vi "File or directory exists.vi"(8 "error in (no error)":errorcluster, 10 "Path":string, 11 "FTP in":refnum<class "FTP.lvclass">) -> (0 "error out":errorcluster, 1 "Exists?":bool, 2 "Path out (dup)":string, 3 "FTP out":refnum<class "FTP.lvclass">, 4 "Type":T1)   [LabVIEW 2015, in "RT Management.lvlib" / "FTP.lvclass"]
uses:
  FTP.lvclass
  File Transfer Behavior/Type.ctl
  FTP.lvclass/FTP.ctl
  Get Session.vi
  <vilib>/Utility/error.llb/Trim Whitespace.vi
  File Transfer Behavior/File Transfer Behavior.lvclass
  <vilib>/FTP/NI_FTP.lvlib
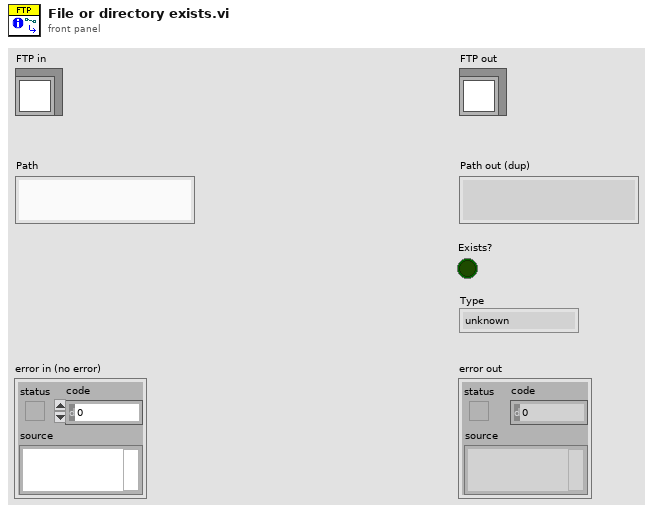
[diagram p1: front panel]
types:
  T1 = typedef "RT Management.lvlib/File Transfer Behavior.lvclass/Type.ctl" = enum16{"unknown", "file", "directory"}
  T2 = typedef "NI_FTP.lvlib/FTP Session.ctl" = refnum<k5>
  T3 = typedef "NI_FTP.lvlib/FTP File Info.ctl" = cluster{"type":enum16{"unknown", "file", "dir", "link"}, "permissions":string, "owner":string, "group":string, "size":i32, "date":string, "name":string, "link name":string}
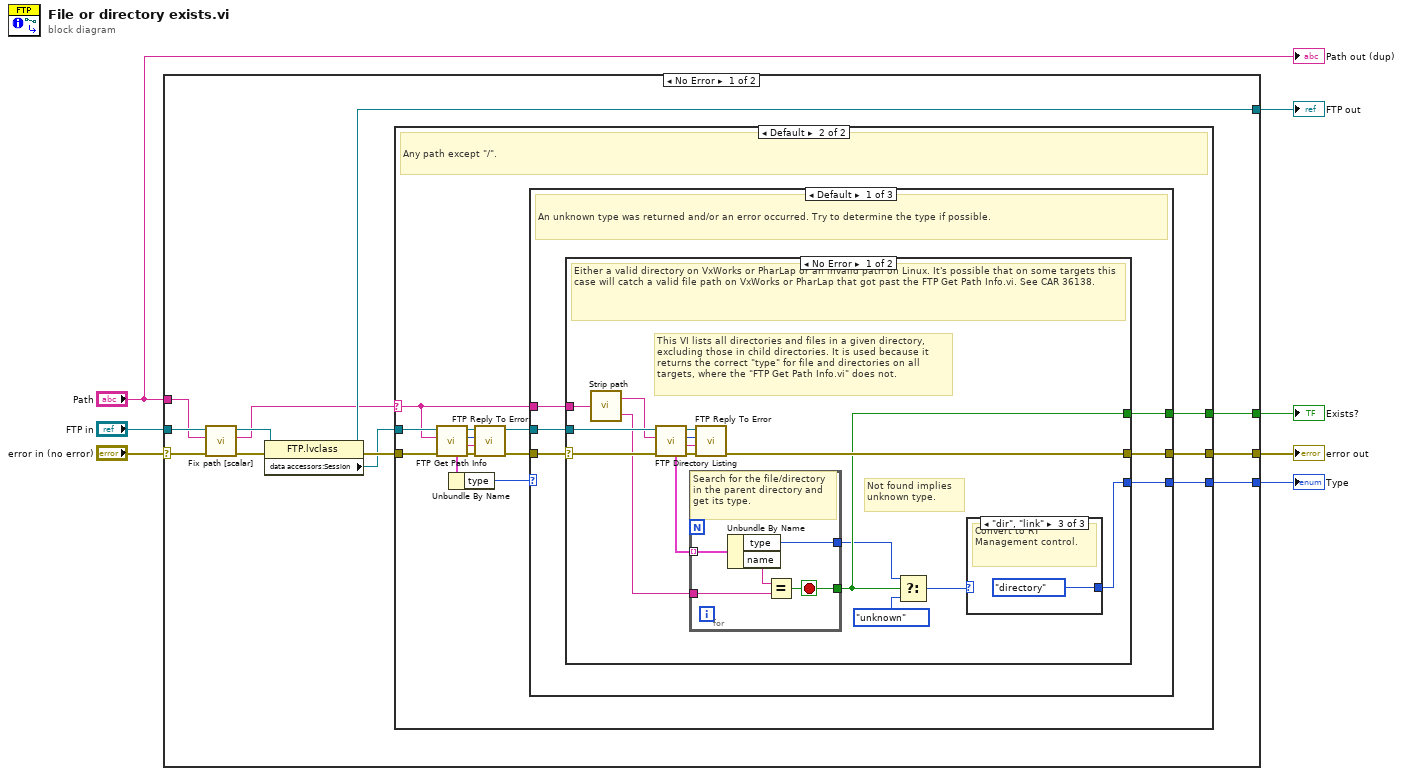
[diagram p0: block diagram]
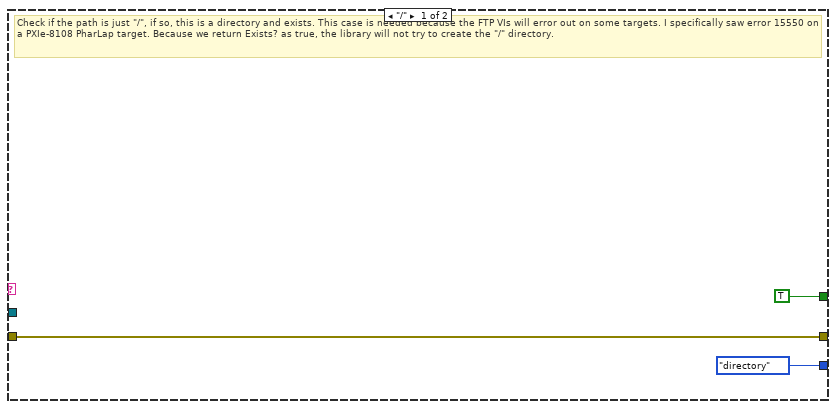
[diagram p2: hidden frame]
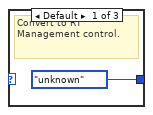
[diagram p3: hidden frame]
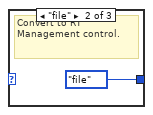
[diagram p4: hidden frame]
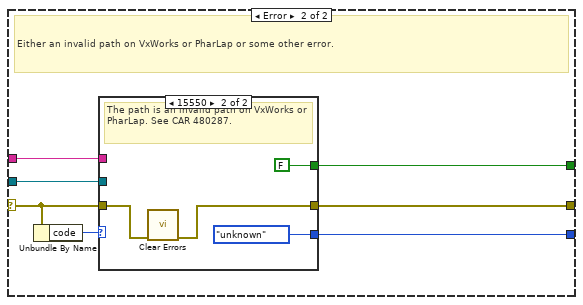
[diagram p5: hidden frame]
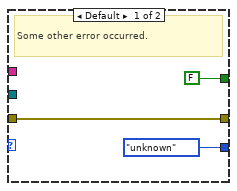
[diagram p6: hidden frame]
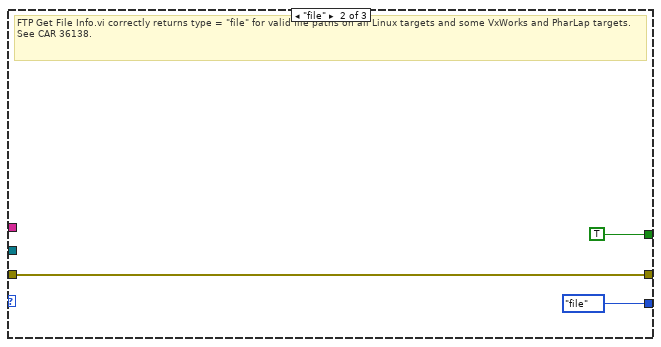
[diagram p7: hidden frame]
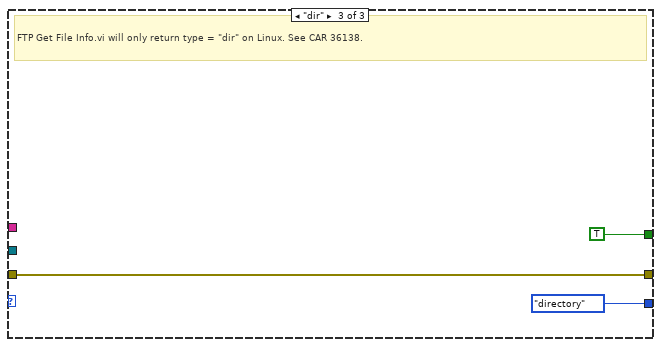
[diagram p8: hidden frame]
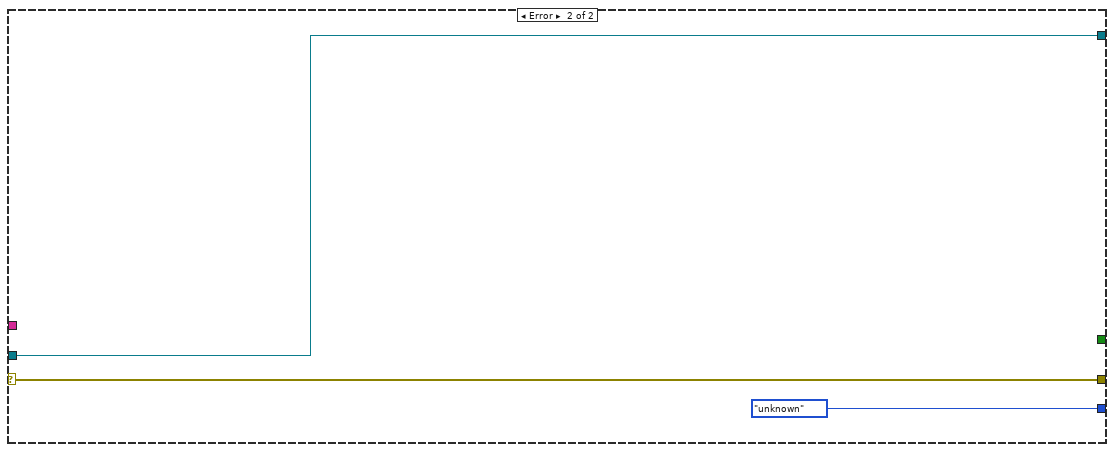
[diagram p9: hidden frame]
diagram:
  n1 = case shown="No Error" "error in (no error)" {
    selector: "error in (no error)" -> [w19 w89]
    tunnel: [w12 w89] -> w6
    tunnel: "FTP in" -> [w18 w88]
    tunnel: [w15 w88] -> w4
    tunnel: "Path" -> [w14 _]
    tunnel: [w11 _] -> w2
    tunnel: [w9 Type."unknown" ("Type")] -> w1
    frame No Error {
      n2 = call "Fix path [scalar].vi"("error in (no error)"=w19, "Path in"=w14, "File Transfer Behavior in"=w18) -> ("error out"=w17:errorcluster, "Path out"=w8:string, "File Transfer Behavior out"=w16:refnum<class "FTP.lvclass">)  [unwired: 6 in]
      n3 = property class="FTP.lvclass"(reference=w16, error in=w17) -> (reference out=w15:refnum<class "FTP.lvclass">, error out=w13:errorcluster, "data accessors:Session"=w10:T2)
      n4 = case shown="Default" w8 {
        selector: w8 -> [_ w23]
        tunnel: w13 -> [w22 w36]
        tunnel: [w22 w34] -> w12
        tunnel: [TRUE w33] -> w11
        tunnel: w10 -> [_ w25]
        tunnel: [Type."directory" ("Type") w24] -> w9
        frame "/" {
          # "Check if the path is just \"/\", if so, this is a directory and exists. This case is needed because the FTP VIs will error out on some targets. I specifically saw error 15550 on a PXIe-8108 PharLap target. Because we return Exists? as true, the library will not try to create the \"/\" directory."
        }
        frame Default {
          # "Any path except \"/\"."
          n5 = call <vilib>:"FTP Get Path Info.vi"("error in (no error)"=w36, "remote path"=w23, "ftp session"=w25) -> ("error out"=w32:errorcluster, "reply string"=w31:string, "reply code"=w30:i32, "ftp session out"=w29:T2, "path info"=w28:T3)  [unwired: 4 in]
          n6 = Unbundle By Name(w28) -> ("type"=w35:enum16{"unknown", "file", "dir", "link"})
          n7 = call <vilib>:"FTP Reply To Error.vi"("error in (no error)"=w32, "reply string in"=w31, "reply code in"=w30, "ftp session"=w29) -> ("error out"=w27:errorcluster, "ftp session out"=w26:T2)  [unwired: 2 out]
          n8 = case shown="Default" w35 {
            tunnel: w27 -> [w38 w82 w85]
            tunnel: [w42 TRUE TRUE] -> w33
            tunnel: w26 -> [w41 _ _]
            tunnel: w23 -> [w40 _ _]
            tunnel: [w39 w82 w85] -> w34
            tunnel: [w37 Type."file" ("Type") Type."directory" ("Type")] -> w24
            frame Default {
              # "An unknown type was returned and/or an error occurred. Try to determine the type if possible."
              n9 = case shown="No Error" w38 {
                selector: w38 -> [w58 w68]
                tunnel: [w54 w72] -> w42
                tunnel: w41 -> [w57 w71]
                tunnel: w40 -> [w56 w70]
                tunnel: [w55 w69] -> w39
                tunnel: [w43 w67] -> w37
                frame No Error {
                  # "Not found implies unknown type."
                  # "This VI lists all directories and files in a given directory, excluding those in child directories. It is used because it returns the correct \"type\" for file and directories on all targets, where the \"FTP Get Path Info.vi\" does not."
                  # "Either a valid directory on VxWorks or PharLap or an invalid path on Linux. It's possible that on some targets this case will catch a valid file path on VxWorks or PharLap that got past the FTP Get Path Info.vi. See CAR 36138."
                  n10 = call "Strip path.vi"("Path"=w56) -> ("Name"=w52:string, "Stripped path"=w45:string)  [unwired: 2 in]
                  n11 = call <vilib>:"FTP Directory Listing.vi"("error in (no error)"=w58, "directory path"=w45, "ftp session"=w57) -> ("error out"=w51:errorcluster, "reply string"=w48:string, "reply code"=w49:i32, "ftp session out"=w50:T2, "dir list"=w53:T3[])  [unwired: 4 in]
                  n12 = for {
                    tunnel: w53 -> [w66] mode=indexing
                    tunnel: [w65] -> w54
                    tunnel: [w64] -> w47
                    tunnel: w52 -> [w63]
                    stop <- w65 stop-if-true
                    # "Search for the file/directory in the parent directory and get its type."
                    n13 = Unbundle By Name(w66) -> ("type"=w64:enum16{"unknown", "file", "dir", "link"}, "name"=w62:string)
                    n14 = Equal?(x=w62, y=w63) -> (x = y?=w65:bool)
                  }
                  n15 = call <vilib>:"FTP Reply To Error.vi"("error in (no error)"=w51, "reply string in"=w48, "reply code in"=w49, "ftp session"=w50) -> ("error out"=w55:errorcluster)  [unwired: 3 out]
                  n16 = Select(t=w47, s=w54, f=enum16{"unknown", "file", "dir", "link"}."unknown") -> (s? t:f=w44:enum16{"unknown", "file", "dir", "link"})
                  n17 = case shown="\"dir\", \"link\"" w44 {
                    tunnel: [Type."unknown" ("Type") Type."file" ("Type") Type."directory" ("Type")] -> w43
                    frame Default {
                      # "Convert to RT Management control."
                    }
                    frame "file" {
                      # "Convert to RT Management control."
                    }
                    frame "dir", "link" {
                      # "Convert to RT Management control."
                    }
                  }
                }
                frame Error {
                  # "Either an invalid path on VxWorks or PharLap or some other error."
                  n18 = Unbundle By Name(w68) -> ("code"=w73:i32)
                  n19 = case shown="15550" w73 {
                    tunnel: w68 -> [w76 w80]
                    tunnel: [FALSE FALSE] -> w72
                    tunnel: w71 -> [_ _]
                    tunnel: [w76 w78] -> w69
                    tunnel: w70 -> [_ _]
                    tunnel: [Type."unknown" ("Type") Type."unknown" ("Type")] -> w67
                    frame Default {
                      # "Some other error occurred."
                    }
                    frame 15550 {
                      # "The path is an invalid path on VxWorks or PharLap. See CAR 480287."
                      n20 = call <vilib>:"Clear Errors.vi"("error in (no error)"=w80) -> ("error out"=w78:errorcluster)  [unwired: 5 in, 1 out]
                    }
                  }
                }
              }
            }
            frame "file" {
              # "FTP Get File Info.vi correctly returns type = \"file\" for valid file paths on all Linux targets and some VxWorks and PharLap targets. See CAR 36138."
            }
            frame "dir" {
              # "FTP Get File Info.vi will only return type = \"dir\" on Linux. See CAR 36138."
            }
          }
        }
      }
    }
    frame Error {
    }
  }
  "error out" <- w6
  "FTP out" <- w4
  "Exists?" <- w2
  "Type" <- w1
  "Path out (dup)" <- "Path"
